vi "IMAQdx Get Session Id.vi"(8 "error in":errorcluster, 11 "Session In":T1) -> (0 "error out":errorcluster, 2 "Session Id":u32 format="%08x", 3 "Session Out":T1)   [LabVIEW 2020, in "NI_Vision_Acquisition_Software.lvlib"]
doc: "Converts a LabVIEW generic refnum to a C Session Id."
uses:
  NI_Vision_Acquisition_Software.lvlib
  IMAQdx.ctl
  niimaqdx.dll
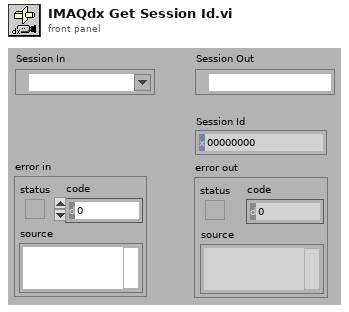
[diagram p1: front panel]
types:
  T1 = typedef "IMAQdx.ctl" = refnum<k21>
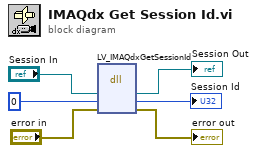
[diagram p0: block diagram]
diagram:
  n1 = dll-call lib="niimaqdx.dll" fn="LV_IMAQdxGetSessionId"("Session In"="Session In", "sessionId"=u32 0 ("driverVersion"), "error in"="error in") -> ("Session In"=→"Session Out":T1, "sessionId"=→"Session Id":u32, "error in"=→"error out":errorcluster)  [unwired: 4 in, 2 out]
